vi "GetFunc.vi"(8 "error in (no error)":errorcluster, 11 "Column in":refnum<class "Column.lvclass">) -> (0 "error out":errorcluster, 1 "isRampable?":bool=TRUE, 2 "isVariable?":bool=TRUE, 3 "Column out":refnum<class "Column.lvclass">, 5 "Disableable?":bool=TRUE)   [LabVIEW 2013, in "Column.lvclass"]
doc: "Initialize functionality booleans (which are never changed).\nIf \"Disableable?\" is set true (false) then certain master modes can(not) prevent the user from changing it's value on a given line. If a column \"isVariable?\" it presents right-click menu items for variables. Both of these are typically TRUE for slave devices.\n\nAlso initialize the approprite \"Num Layouts\" if passed number > 0. For Num Layouts < 1, just pass through whatever layouts exist."
uses:
  Column.lvclass
  Column.lvclass/Column.ctl
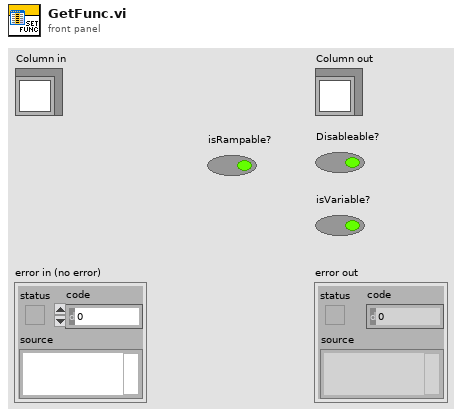
[diagram p1: front panel]
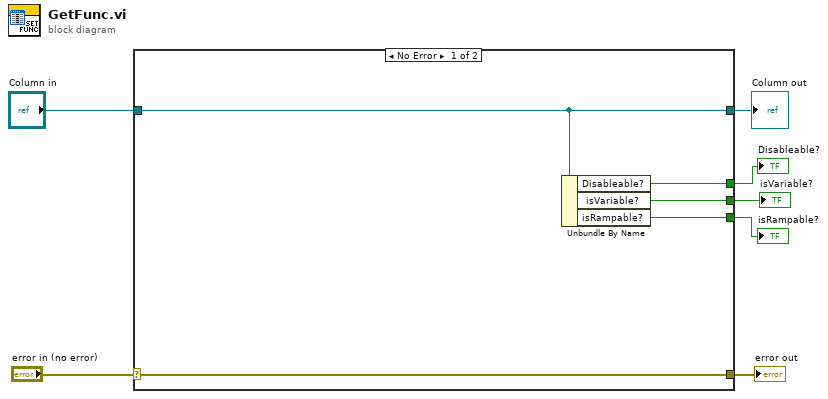
[diagram p0: block diagram]
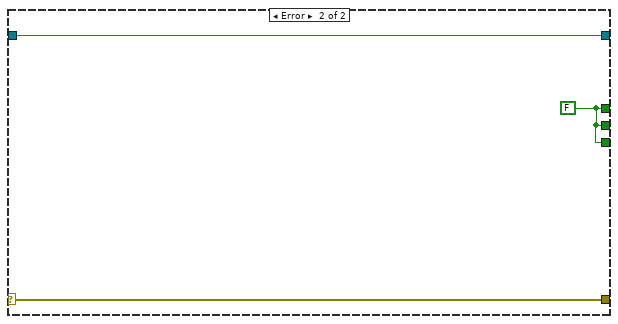
[diagram p2: hidden frame]
diagram:
  n1 = case shown="No Error" "error in (no error)" {
    selector: "error in (no error)" -> [w11 w15]
    tunnel: [w11 w15] -> w6
    tunnel: [w12 w14] -> w4
    tunnel: "Column in" -> [w12 w14]
    tunnel: [w10 w13] -> w3
    tunnel: [w9 w13] -> w2
    tunnel: [w8 w13] -> w1
    frame No Error {
      n2 = Unbundle By Name(w12) -> ("Disableable?"=w10:bool, "isVariable?"=w9:bool, "isRampable?"=w8:bool)
    }
    frame Error {
      w13 = FALSE ("Disableable?")
    }
  }
  "error out" <- w6
  "Column out" <- w4
  "Disableable?" <- w3
  "isVariable?" <- w2
  "isRampable?" <- w1
